vi "IMAQdx_Cam4.vi"(0 "Ctl Ref Record":refnum<vi>, 1 "Ctl Ref Cam":refnum<vi>, 2 "Session In":T6, 3 "Ctl Ref Folder":refnum<vi>, 5 "Cluster Buffer":T1={"Number of Images"=30, "Number of Workers"=5, "Skip Count"=0} {"Number of Workers" min=1 max=5}, 7 "Ctl Ref Time":refnum<vi>, 9 "Ctl Ref WriteSpeed":refnum<vi>, 11 "Ctl Ref Frames":refnum<vi>, 13 "Ctl Ref Stop":refnum<vi>) -> ()   [LabVIEW 2020]
uses:
  <vilib>/vision/driver/IMAQdx.llb/IMAQdx Acquisition Mode.ctl
  <vilib>/vision/Image Controls.llb/IMAQ Image.ctl
  <vilib>/vision/driver/IMAQdx.llb/IMAQdx Buffer Number Mode.ctl
  <vilib>/Utility/High Resolution Relative Seconds.vi
  <vilib>/functionblocks/Edge Detection/One Shot Rising with Input/One Shot Rising with Input.vi
  <vilib>/functionblocks/FB Core/FB Core.xnode
  <vilib>/vision/driver/NI_Vision_Acquisition_Software.lvlib
  <resource>/objmgr/imaqdx.rc
  <vilib>/functionblocks/NI_FunctionBlock Libraries.lvlib
panel:
  out "Cluster Frames":T2
  out "Cluster WriteSpeed":T3 {"WriteSpeed Worker5" format="%_19f"; "WriteSpeed Worker4" format="%_19f"; "WriteSpeed Worker3" format="%_19f"; "WriteSpeed Worker2" format="%_19f"; "WriteSpeed Worker1" format="%_19f"}
  out "Cluster BufferNr":T4
  out "Cluster LoopTimer":T5
  in  "Recording":bool
  out "VideoMode Camera":u32[](array[numeric])
  out "VideoMode Camera":string[](array[string])
  in  "Stop":bool
  out "Images in Queue":i32
  out "Camera":T7(plugin-control)
  out "LostBufferCount":u32
  out "Destination Folder":path
  in  "Stopped":bool
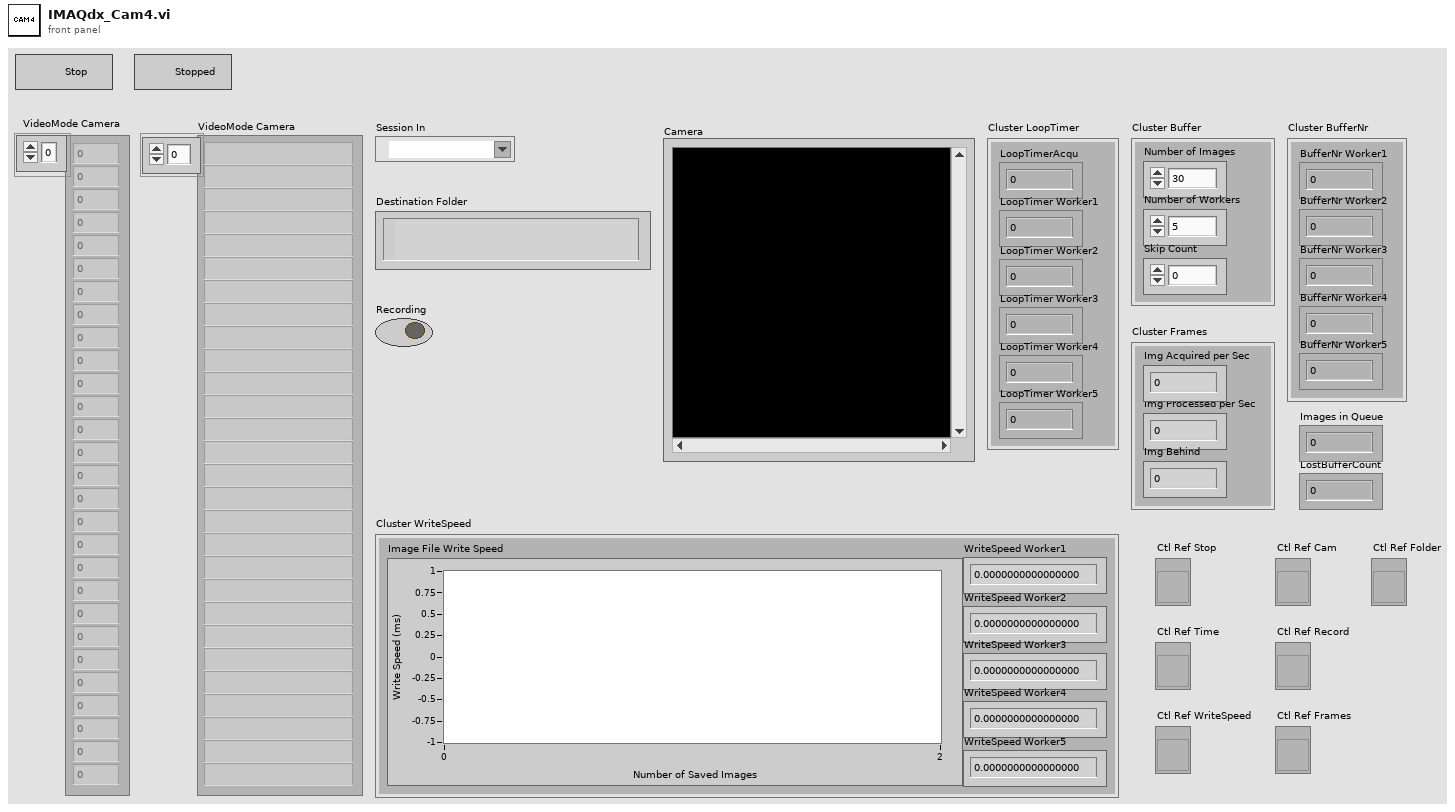
[diagram p1: front panel]
types:
  T1 = cluster{"Number of Images":i32, "Number of Workers":u8, "Skip Count":u32}
  T2 = cluster{"Img Processed per Sec":dbl, "Img Behind":i32, "Img Acquired per Sec":dbl}
  T3 = cluster{"WriteSpeed Worker1":dbl, "WriteSpeed Worker2":dbl, "WriteSpeed Worker3":dbl, "WriteSpeed Worker4":dbl, "WriteSpeed Worker5":dbl, "Write Speed":dbl}
  T4 = cluster{"BufferNr Worker1":u32, "BufferNr Worker2":u32, "BufferNr Worker3":u32, "BufferNr Worker4":u32, "BufferNr Worker5":u32}
  T5 = cluster{"LoopTimerAcqu":u32, "LoopTimer Worker1":u32, "LoopTimer Worker2":u32, "LoopTimer Worker3":u32, "LoopTimer Worker4":u32, "LoopTimer Worker5":u32}
  T6 = typedef "IMAQdx.ctl" = refnum<k21>
  T7 = typedef "IMAQ Image.ctl" = refnum<image>
  T8 = cluster{"Image Out":T7, "Buffer Number Out":u32, string}
  T9 = typedef "NI_Vision_Acquisition_Software.lvlib/IMAQdx Acquisition Mode.ctl" = enum32{"One Shot", "Continuous"}
  T10 = cluster{"Video Mode":u32, "Video Mode Name":string}[]
  T11 = typedef "NI_Vision_Acquisition_Software.lvlib/IMAQdx Buffer Number Mode.ctl" = enum32{"Next", "Last", "Buffer Number", "Every", "Last New"}
  T12 = cluster{"Image Out":T7, "Buffer Number Out":u32, "date/time string":string}
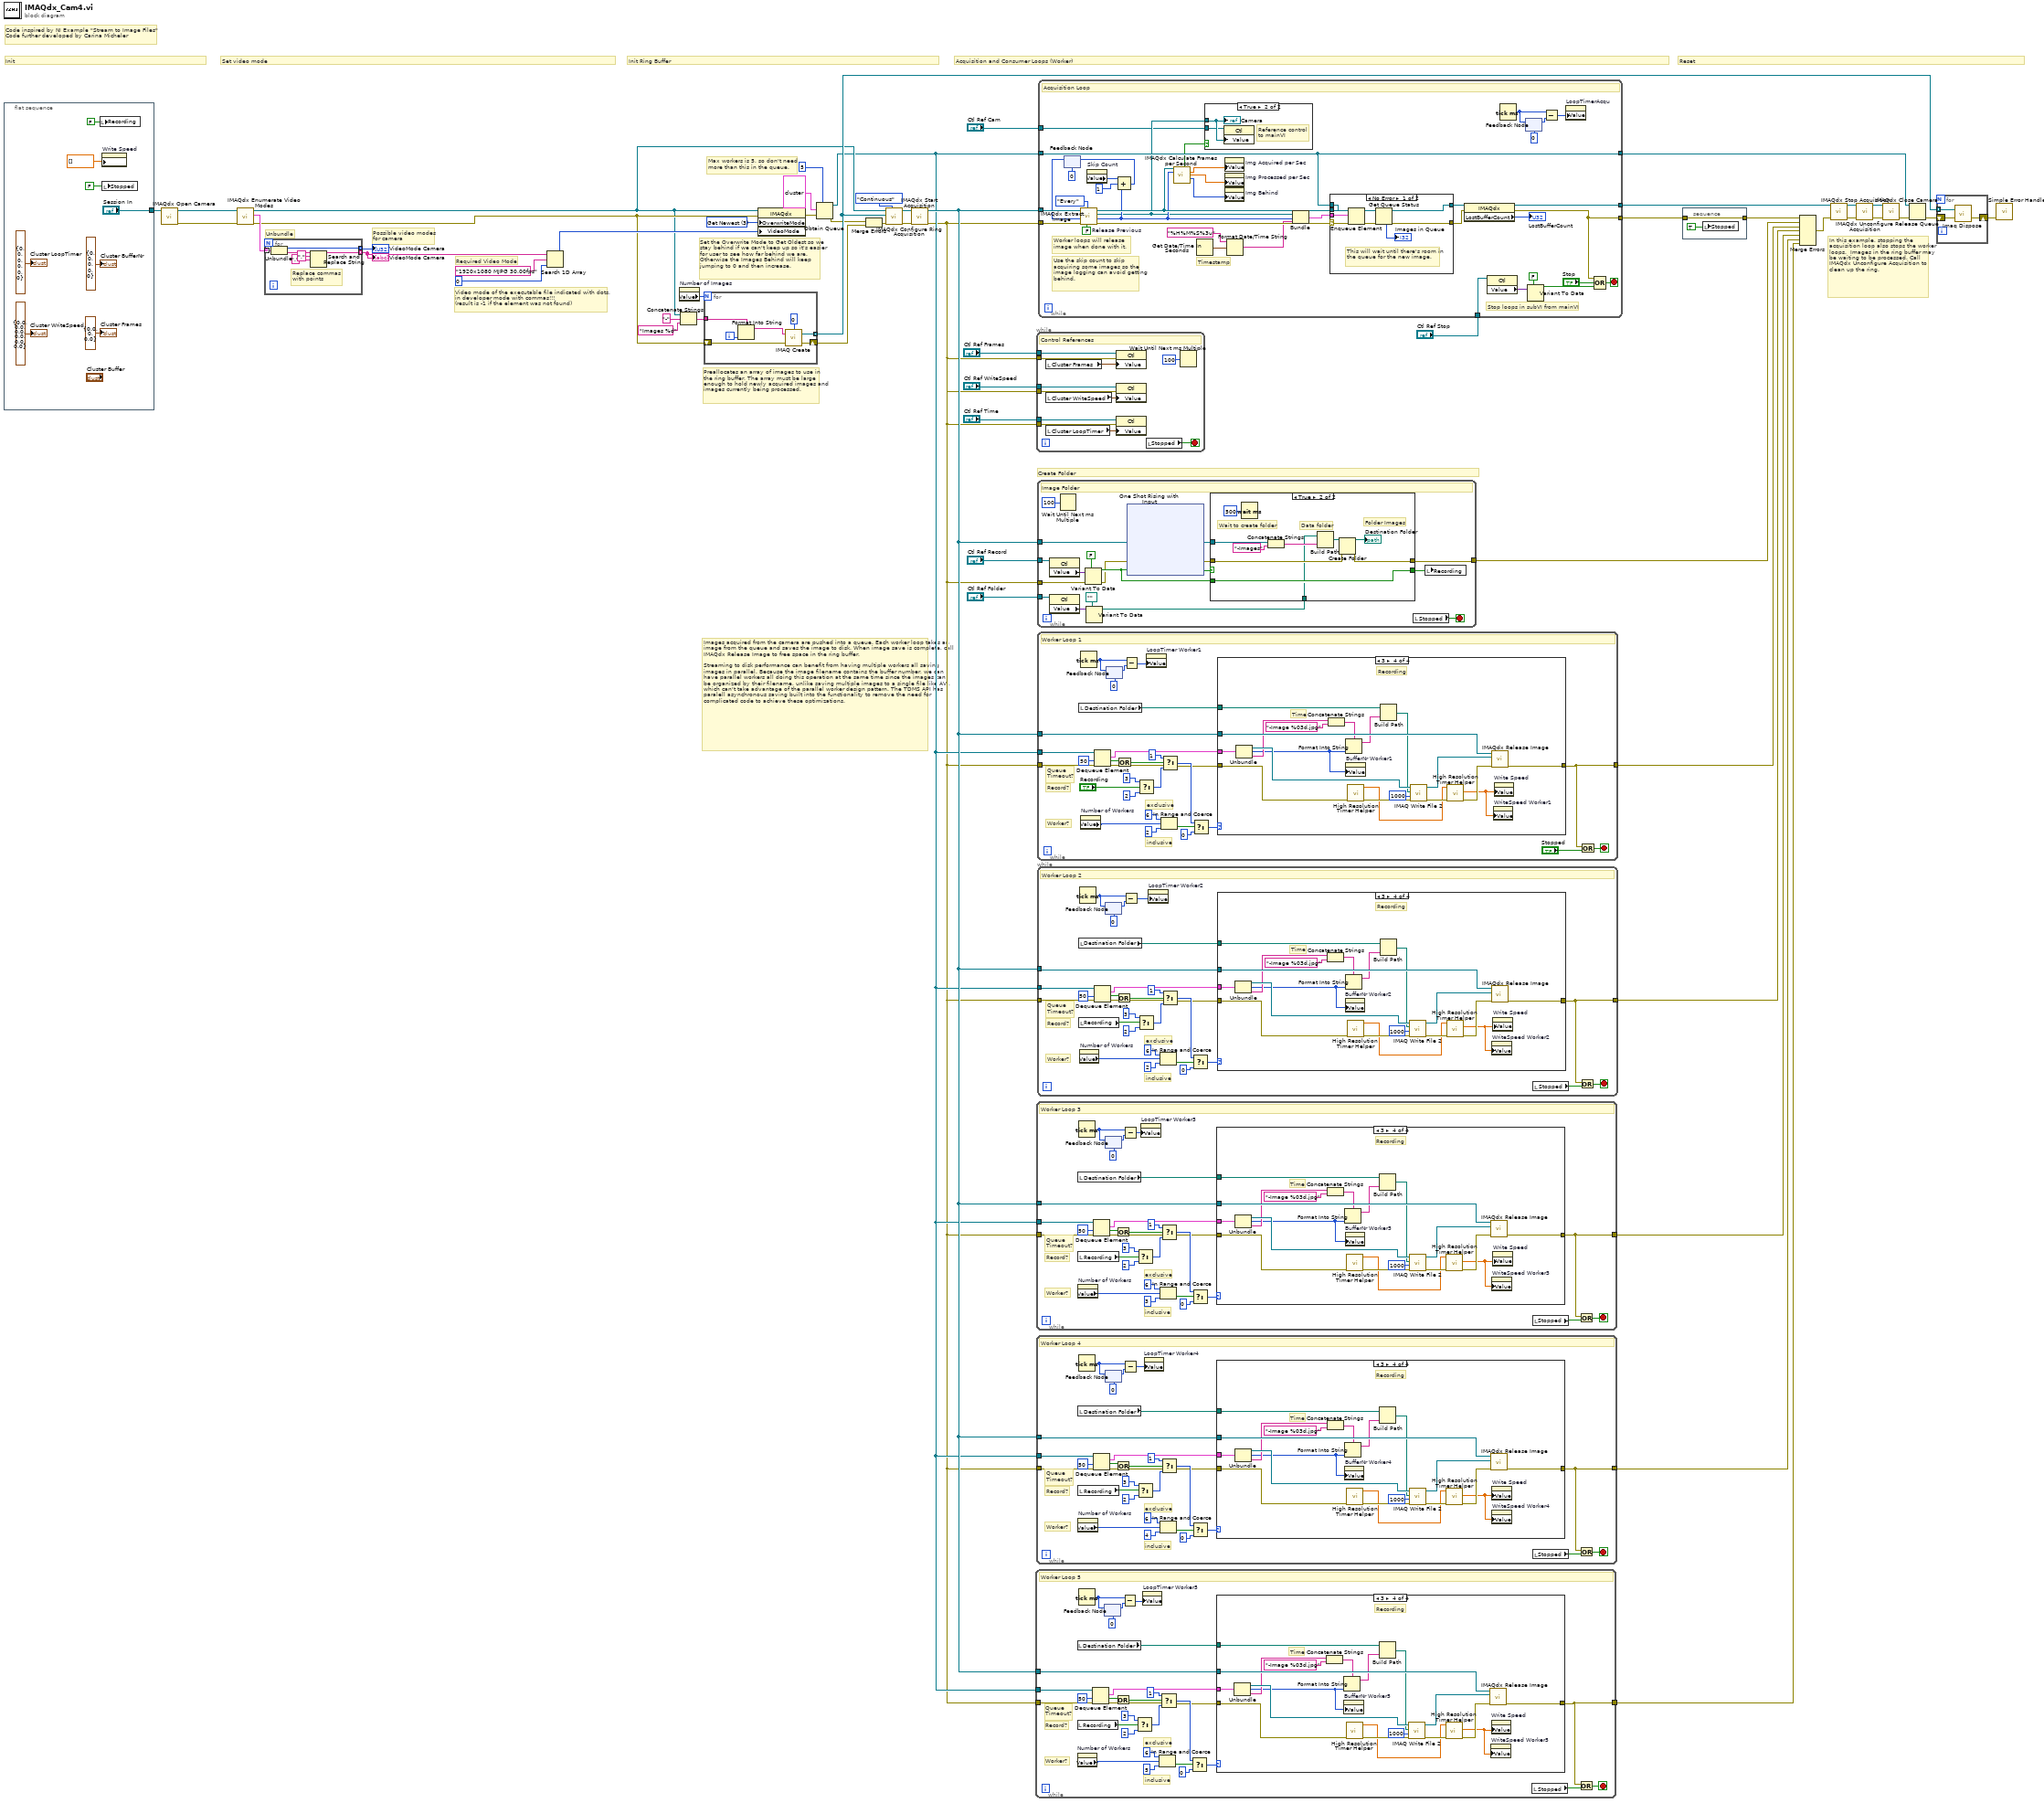
[diagram p0: block diagram]
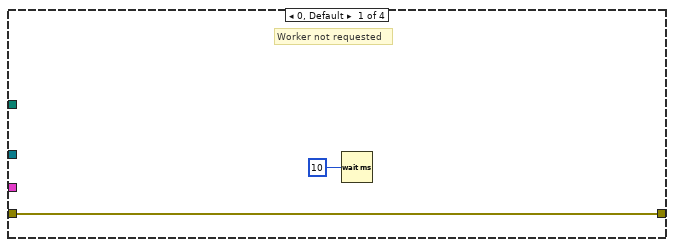
[diagram p2: hidden frame]
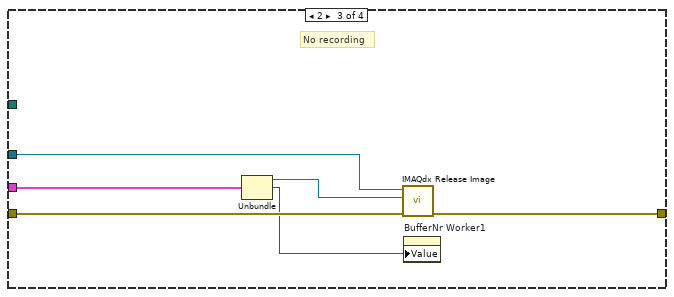
[diagram p4: hidden frame]
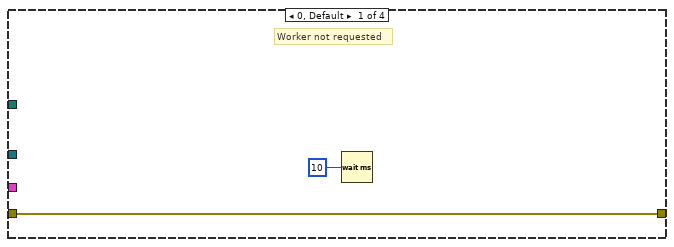
[diagram p5: hidden frame]
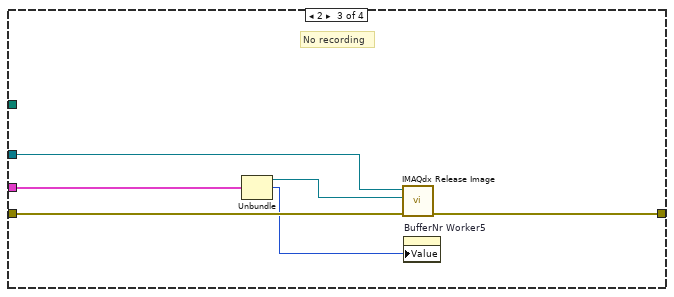
[diagram p7: hidden frame]
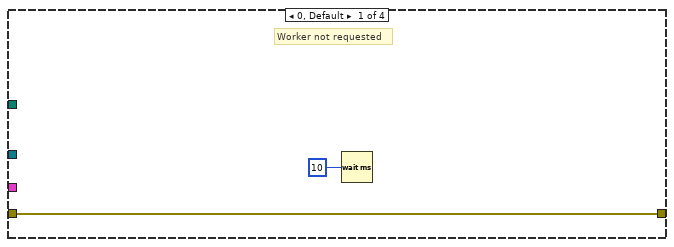
[diagram p8: hidden frame]
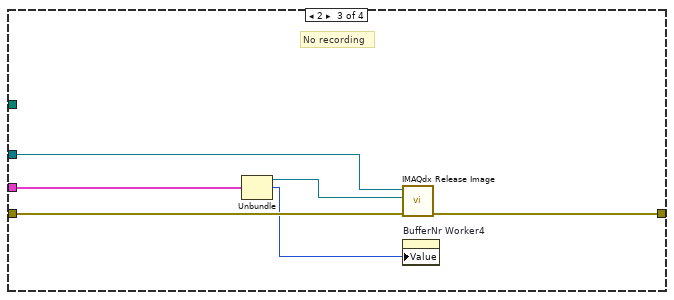
[diagram p10: hidden frame]
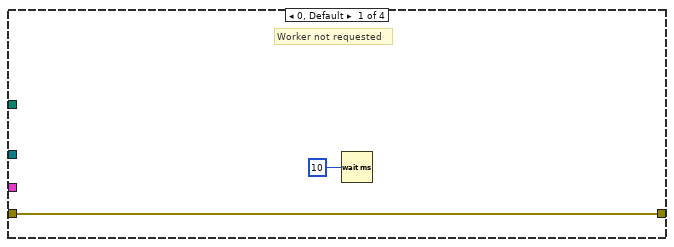
[diagram p11: hidden frame]
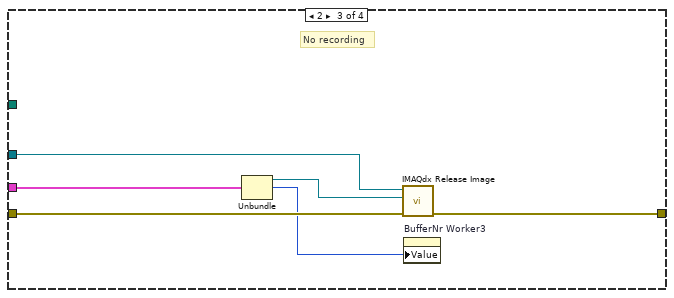
[diagram p13: hidden frame]
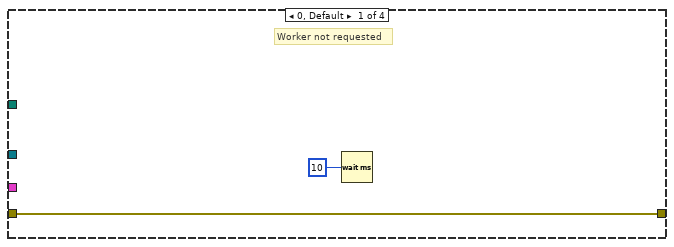
[diagram p15: hidden frame]
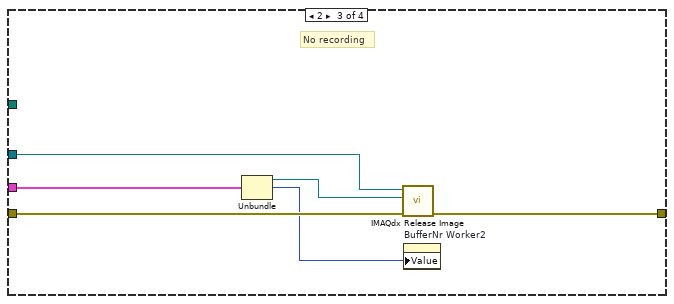
[diagram p17: hidden frame]
diagram:
  w35 = u32 3 items=["Get Oldest"=0, "Fail"=2, "Get Newest"=3] ("OverwriteMode")
  # "Create Folder"
  # "Images acquired from the camera are pushed into a queue. Each worker loop takes an image from the queue and saves the image to disk. When image save is complete, call IMAQdx Release Image to free space in the ring buffer. \n\nStreaming to disk performance can benefit from having multiple workers all saving images in parallel. Because the image filename contains the buffer number, we can have parallel workers all doing this operation at the same time since the images can be organized by their filename, unlike saving multiple images to a single file like AVI, which can't take advantage of the parallel worker design pattern. The TDMS API has paralell asynchronous saving built into the functionality to remove the need for complicated code to achieve these optimizations."
  # "Acquisition and Consumer Loops (Worker)"
  # "Reset"
  # "Code inspired by NI Example \"Stream to Image Files\"\nCode further developed by Carina Micheler"
  # "Init Ring Buffer"
  # "Init"
  # "Set video mode"
  # "Video mode of the executable file indicated with dots,\nin developer mode with commas!!!\n(result is -1 if the element was not found)"
  # "Required Video Mode"
  # "Possible video modes\nfor camera"
  # "Unbundle"
  # "Set the Overwrite Mode to Get Oldest so we stay behind if we can't keep up so it's easier for user to see how far behind we are. Otherwise the Images Behind will keep jumping to 0 and then increase."
  # "Max workers is 5, so don't need more than this in the queue."
  # "In this example, stopping the acquisition loop also stops the worker loops.  Images in the ring buffer may be waiting to be processed. Call IMAQdx Unconfigure Acquisition to clean up the ring."
  # "Preallocates an array of images to use in the ring buffer. The array must be large enough to hold newly acquired images and images currently being processed."
  n1 = flat-sequence {
    tunnel: ["Session In"] -> w22
    frame #0 {
      n2 = local write "Recording"(FALSE ("Recording")) -> ()
      n3 = property on="Write Speed" class="WFChart (strict)"("History Data"=dbl[] []) -> ()  [unwired: 2 in, 2 out]
      n4 = local write "Stopped"(FALSE ("Stop")) -> ()
      "Cluster LoopTimer" <- T5 {"LoopTimerAcqu"=0, "LoopTimer Worker1"=0, "LoopTimer Worker2"=0, "LoopTimer Worker3"=0, "LoopTimer Worker4"=0, "LoopTimer Worker5"=0} ("Cluster LoopTimer")
      "Cluster BufferNr" <- T4 {"BufferNr Worker1"=0, "BufferNr Worker2"=0, "BufferNr Worker3"=0, "BufferNr Worker4"=0, "BufferNr Worker5"=0} ("Cluster BufferNr")
      "Cluster WriteSpeed" <- T3 {"WriteSpeed Worker1"=0.0, "WriteSpeed Worker2"=0.0, "WriteSpeed Worker3"=0.0, "WriteSpeed Worker4"=0.0, "WriteSpeed Worker5"=0.0, "Write Speed"=0.0} ("Cluster WriteSpeed")
      "Cluster Frames" <- T2 {"Img Processed per Sec"=0.0, "Img Behind"=0, "Img Acquired per Sec"=0.0} ("Cluster Frames")
    }
  }
  n5 = call <vilib>:"IMAQdx Open Camera.vi"("Session In"=w22) -> ("error out"=w23:errorcluster, "Session Out"=w24:T6)  [unwired: 2 in, 7 out]
  n6 = call <vilib>:"IMAQdx Enumerate Video Modes.vi"("error in"=w23, "Session In"=w24) -> ("error out"=w25:errorcluster, "Video Modes"=w31:T10, "Session Out"=w15:T6)  [unwired: 6 in, 1 out]
  n7 = for {
    tunnel: w31 -> [w68] mode=indexing
    tunnel: [w67] -> w29 mode=indexing
    tunnel: [w63] -> w30 mode=indexing
    # "Replace commas \nwith points"
    n8 = Unbundle(w68) -> ("Video Mode"=w67:u32, "Video Mode Name"=w66:string)
    n9 = Search and Replace String(input string=w66, search string=",", replace string="." ("replace string (\"\")")) -> (result string=w63:string)  [unwired: 5 in, 3 out]
  }
  "VideoMode Camera" <- w30
  "VideoMode Camera" <- w29
  n10 = Search 1D Array(1D array=w30, element="1920x1080 MJPG 30.00fps", start index (0)=0) -> (index of element=w26:i32)
  n11 = property on="Number of Images" class="DigNum (strict)"() -> ("Value"=w7:i32)  [unwired: 2 in, 2 out]
  n12 = Concatenate Strings(w15, "-" ("string"), "Images %d" ("Image Name")) -> (w18:string)
  n13 = for {
    N: w7 -> [_]
    tunnel: [w74] -> w43 mode=indexing
    shift-right: [w73] -> w21
    shift-left: w25 -> [w75]
    tunnel: w18 -> [w69]
    i -> [w72]
    n14 = Format Into String(format string=w69, w72) -> (resulting string=w70:string)  [unwired: 2 in, 1 out]
    n15 = call "IMAQ Create"("Border Size"=0, "Image Name"=w70, "error in (no error)"=w75) -> ("New Image"=w74:T7, "error out"=w73:errorcluster)  [unwired: 1 in, 1 out]
  }
  n16 = property class="IMAQdx"(reference=w15, error in=w25, "OverwriteMode"=w35, "VideoMode"=w26) -> (error out=w34:errorcluster)  [unwired: 1 out]
  n17 = Obtain Queue(max queue size (-1, unlimited)=5, element data type=T8 {"Image Out"=refnum, "Buffer Number Out"=0, ""}, error in (no error)=w34) -> (queue out=w9:refnum<queue>, error out=w33:errorcluster)  [unwired: 2 in, 1 out]
  n18 = Merge Errors(w33, w21) -> (w46:errorcluster)
  n19 = call <vilib>:"IMAQdx Configure Ring Acquisition.vi"("Mode"=IMAQdx_Acquisition_Mode."Continuous" ("Continuous?"), "error in"=w46, "Images"=w43, "Session In"=w15) -> ("error out"=w49:errorcluster, "Session Out"=w50:T6)  [unwired: 5 in, 1 out]
  n20 = call <vilib>:"IMAQdx Start Acquisition.vi"("error in"=w49, "Session In"=w50) -> ("error out"=w3:errorcluster, "Session Out"=w10:T6)  [unwired: 8 out]
  n21 = while {
    tunnel: w9 -> [w80]
    tunnel: w10 -> [w102]
    tunnel: w3 -> [w82]
    tunnel: [w101] -> w11
    stop <- w103 stop-if-true
    # "Queue \nTimeout?"
    # "Record?"
    # "Worker?"
    # "inclusive"
    # "exclusive"
    # "Worker Loop 5"
    n22 = local read "Destination Folder"() -> (w99:path)
    n23 = local read "Recording"() -> (w93:bool)
    n24 = property on="Number of Workers" class="DigNum (strict)"() -> ("Value"=w76:u8)  [unwired: 2 in, 2 out]
    n25 = Tick Count (ms)() -> (millisecond timer value=w98:u32)
    n26 = Dequeue Element(queue=w80, timeout in ms (-1)=50 ("timeout in ms"), error in (no error)=w82) -> (element=w79:T8, timed out?=w90:bool, error out=w81:errorcluster)  [unwired: 1 out]
    n27 = feedback #1(u32 0 ("millisecond timer value")) -> (w97:u32)
    n28 = feedback-in #1(w98) -> ()
    n29 = Or(x=w90, y=w81) -> (x .or. y?=w92:bool)
    n30 = Subtract(x=w98, y=w97) -> (x-y=w77:u32)
    n31 = Select(t=u8 3 ("y"), s=w93, f=u8 2 ("y")) -> (s? t:f=w94:u8)
    n32 = property on="LoopTimer Worker5" class="DigNum (strict)"("Value"=w77) -> ()  [unwired: 2 in, 2 out]
    n33 = In Range and Coerce(upper limit=u8 6 ("y"), x=w76, lower limit=u8 5 ("y")) -> (In Range?=w95:bool)  [unwired: 1 out]
    n34 = Select(t=u8 1 ("y"), s=w92, f=w94) -> (s? t:f=w91:u8)
    n35 = Select(t=w91, s=w95, f=u8 0 ("y")) -> (s? t:f=w83:u8)
    n36 = case shown="3" w83 {
      tunnel: w102 -> [_ _ w112 w131]
      tunnel: w99 -> [_ _ _ w130]
      tunnel: w81 -> [w105 w106 w109 w128]
      tunnel: [w105 w106 w111 w129] -> w101
      tunnel: w79 -> [_ _ w110 w127]
      frame 0, Default {
        # "Worker not requested"
        n37 = Wait (ms)(milliseconds to wait=u32 10) -> ()  [unwired: 1 out]
      }
      frame 1 {
        # "Empty queue or error.\nNothing to process."
      }
      frame 2 {
        # "No recording"
        n38 = Unbundle(w110) -> ("Image Out"=w108:T7, "Buffer Number Out"=w107:u32)  [unwired: 1 out]
        n39 = call <vilib>:"IMAQdx Release Image.vi"("error in"=w109, "Image"=w108, "Session In"=w112) -> ("error out"=w111:errorcluster)  [unwired: 7 in, 1 out]
        n40 = property on="BufferNr Worker5" class="DigNum (strict)"("Value"=w107) -> ()  [unwired: 2 in, 2 out]
      }
      frame 3 {
        # "Recording"
        # "Time"
        n41 = Unbundle(w127) -> ("Image Out"=w126:T7, "Buffer Number Out"=w114:u32, w119:string)
        n42 = Concatenate Strings(w119, "-Image %03d.jpg" ("format string")) -> (w121:string)
        n43 = Format Into String(format string=w121, w114) -> (resulting string=w124:string)  [unwired: 2 in, 1 out]
        n44 = property on="BufferNr Worker5" class="DigNum (strict)"("Value"=w114) -> ()  [unwired: 2 in, 2 out]
        n45 = call "High Resolution Timer Helper.vi"("error in (no error)"=w128) -> ("error out"=w118:errorcluster, "Current Time"=w116:dbl)  [unwired: 8 in, 1 out]
        n46 = Build Path(base path=w130, name or relative path=w124) -> (appended path=w123:path)
        n47 = call-poly "IMAQ Write File 2"("error in (no error)"=w118, "Image Quality"=u32 1000, "File Path"=w123, "Image"=w126) -> ("error out"=w117:errorcluster, "Image Out (duplicate)"=w125:T7)  [unwired: 6 in]
        n48 = call "High Resolution Timer Helper.vi"("error in (no error)"=w117, "Previous Time"=w116) -> ("error out"=w122:errorcluster, "Time Difference (ms)"=w113:dbl)  [unwired: 7 in, 1 out]
        n49 = call <vilib>:"IMAQdx Release Image.vi"("error in"=w122, "Image"=w125, "Session In"=w131) -> ("error out"=w129:errorcluster)  [unwired: 7 in, 1 out]
        n50 = property on="WriteSpeed Worker5" class="DigNum (strict)"("Value"=w113) -> ()  [unwired: 2 in, 2 out]
        n51 = property on="Write Speed" class="WFChart (strict)"("Value"=w113) -> ()  [unwired: 2 in, 2 out]
      }
    }
    n52 = local read "Stopped"() -> (w100:bool)
    n53 = Or(x=w101, y=w100) -> (x .or. y?=w103:bool)
  }
  n54 = while {
    tunnel: "Ctl Ref Time" -> [w141]
    tunnel: w3 -> [w139]
    tunnel: "Ctl Ref WriteSpeed" -> [w136]
    tunnel: w3 -> [w137]
    tunnel: "Ctl Ref Frames" -> [w134]
    tunnel: w3 -> [w133]
    stop <- w140 stop-if-true
    # "Control References"
    n55 = local read "Cluster Frames"() -> (w132:T2)
    n56 = local read "Cluster WriteSpeed"() -> (w135:T3)
    n57 = local read "Cluster LoopTimer"() -> (w142:T5)
    n58 = property class="Ctl"(reference=w134, error in=w133, "Value"=w132) -> ()  [unwired: 2 out]
    n59 = property class="Ctl"(reference=w136, error in=w137, "Value"=w135) -> ()  [unwired: 2 out]
    n60 = property class="Ctl"(reference=w141, error in=w139, "Value"=w142) -> ()  [unwired: 2 out]
    n61 = local read "Stopped"() -> (w140:bool)
    n62 = Wait Until Next ms Multiple(millisecond multiple=u32 100) -> ()  [unwired: 1 out]
  }
  n63 = while {
    tunnel: w9 -> [w147]
    tunnel: w10 -> [w169]
    tunnel: w3 -> [w149]
    tunnel: [w168] -> w13
    stop <- w170 stop-if-true
    # "Queue \nTimeout?"
    # "Record?"
    # "Worker?"
    # "inclusive"
    # "exclusive"
    # "Worker Loop 3"
    n64 = local read "Destination Folder"() -> (w166:path)
    n65 = local read "Recording"() -> (w160:bool)
    n66 = property on="Number of Workers" class="DigNum (strict)"() -> ("Value"=w143:u8)  [unwired: 2 in, 2 out]
    n67 = Tick Count (ms)() -> (millisecond timer value=w165:u32)
    n68 = Dequeue Element(queue=w147, timeout in ms (-1)=50 ("timeout in ms"), error in (no error)=w149) -> (element=w146:T8, timed out?=w157:bool, error out=w148:errorcluster)  [unwired: 1 out]
    n69 = feedback #2(u32 0 ("millisecond timer value")) -> (w164:u32)
    n70 = feedback-in #2(w165) -> ()
    n71 = Or(x=w157, y=w148) -> (x .or. y?=w159:bool)
    n72 = Subtract(x=w165, y=w164) -> (x-y=w144:u32)
    n73 = Select(t=u8 3 ("y"), s=w160, f=u8 2 ("y")) -> (s? t:f=w161:u8)
    n74 = property on="LoopTimer Worker3" class="DigNum (strict)"("Value"=w144) -> ()  [unwired: 2 in, 2 out]
    n75 = In Range and Coerce(upper limit=u8 6 ("y"), x=w143, lower limit=u8 3 ("y")) -> (In Range?=w162:bool)  [unwired: 1 out]
    n76 = Select(t=u8 1 ("y"), s=w159, f=w161) -> (s? t:f=w158:u8)
    n77 = Select(t=w158, s=w162, f=u8 0 ("y")) -> (s? t:f=w150:u8)
    n78 = case shown="3" w150 {
      tunnel: w169 -> [_ _ w179 w198]
      tunnel: w166 -> [_ _ _ w197]
      tunnel: w148 -> [w172 w173 w176 w195]
      tunnel: [w172 w173 w178 w196] -> w168
      tunnel: w146 -> [_ _ w177 w194]
      frame 0, Default {
        # "Worker not requested"
        n79 = Wait (ms)(milliseconds to wait=u32 10) -> ()  [unwired: 1 out]
      }
      frame 1 {
        # "Empty queue or error.\nNothing to process."
      }
      frame 2 {
        # "No recording"
        n80 = Unbundle(w177) -> ("Image Out"=w175:T7, "Buffer Number Out"=w174:u32)  [unwired: 1 out]
        n81 = call <vilib>:"IMAQdx Release Image.vi"("error in"=w176, "Image"=w175, "Session In"=w179) -> ("error out"=w178:errorcluster)  [unwired: 7 in, 1 out]
        n82 = property on="BufferNr Worker3" class="DigNum (strict)"("Value"=w174) -> ()  [unwired: 2 in, 2 out]
      }
      frame 3 {
        # "Recording"
        # "Time"
        n83 = Unbundle(w194) -> ("Image Out"=w193:T7, "Buffer Number Out"=w181:u32, w186:string)
        n84 = Concatenate Strings(w186, "-Image %03d.jpg" ("format string")) -> (w188:string)
        n85 = Format Into String(format string=w188, w181) -> (resulting string=w191:string)  [unwired: 2 in, 1 out]
        n86 = property on="BufferNr Worker3" class="DigNum (strict)"("Value"=w181) -> ()  [unwired: 2 in, 2 out]
        n87 = call "High Resolution Timer Helper.vi"("error in (no error)"=w195) -> ("error out"=w185:errorcluster, "Current Time"=w183:dbl)  [unwired: 8 in, 1 out]
        n88 = Build Path(base path=w197, name or relative path=w191) -> (appended path=w190:path)
        n89 = call-poly "IMAQ Write File 2"("error in (no error)"=w185, "Image Quality"=u32 1000, "File Path"=w190, "Image"=w193) -> ("error out"=w184:errorcluster, "Image Out (duplicate)"=w192:T7)  [unwired: 6 in]
        n90 = call "High Resolution Timer Helper.vi"("error in (no error)"=w184, "Previous Time"=w183) -> ("error out"=w189:errorcluster, "Time Difference (ms)"=w180:dbl)  [unwired: 7 in, 1 out]
        n91 = call <vilib>:"IMAQdx Release Image.vi"("error in"=w189, "Image"=w192, "Session In"=w198) -> ("error out"=w196:errorcluster)  [unwired: 7 in, 1 out]
        n92 = property on="WriteSpeed Worker3" class="DigNum (strict)"("Value"=w180) -> ()  [unwired: 2 in, 2 out]
        n93 = property on="Write Speed" class="WFChart (strict)"("Value"=w180) -> ()  [unwired: 2 in, 2 out]
      }
    }
    n94 = local read "Stopped"() -> (w167:bool)
    n95 = Or(x=w168, y=w167) -> (x .or. y?=w170:bool)
  }
  n96 = while {
    tunnel: w9 -> [w203]
    tunnel: w10 -> [w225]
    tunnel: w3 -> [w205]
    tunnel: [w224] -> w12
    stop <- w226 stop-if-true
    # "Queue \nTimeout?"
    # "Record?"
    # "Worker?"
    # "inclusive"
    # "exclusive"
    # "Worker Loop 4"
    n97 = local read "Destination Folder"() -> (w222:path)
    n98 = local read "Recording"() -> (w216:bool)
    n99 = property on="Number of Workers" class="DigNum (strict)"() -> ("Value"=w199:u8)  [unwired: 2 in, 2 out]
    n100 = Tick Count (ms)() -> (millisecond timer value=w221:u32)
    n101 = Dequeue Element(queue=w203, timeout in ms (-1)=50 ("timeout in ms"), error in (no error)=w205) -> (element=w202:T8, timed out?=w213:bool, error out=w204:errorcluster)  [unwired: 1 out]
    n102 = feedback #3(u32 0 ("millisecond timer value")) -> (w220:u32)
    n103 = feedback-in #3(w221) -> ()
    n104 = Or(x=w213, y=w204) -> (x .or. y?=w215:bool)
    n105 = Subtract(x=w221, y=w220) -> (x-y=w200:u32)
    n106 = Select(t=u8 3 ("y"), s=w216, f=u8 2 ("y")) -> (s? t:f=w217:u8)
    n107 = property on="LoopTimer Worker4" class="DigNum (strict)"("Value"=w200) -> ()  [unwired: 2 in, 2 out]
    n108 = In Range and Coerce(upper limit=u8 6 ("y"), x=w199, lower limit=u8 4 ("y")) -> (In Range?=w218:bool)  [unwired: 1 out]
    n109 = Select(t=u8 1 ("y"), s=w215, f=w217) -> (s? t:f=w214:u8)
    n110 = Select(t=w214, s=w218, f=u8 0 ("y")) -> (s? t:f=w206:u8)
    n111 = case shown="3" w206 {
      tunnel: w225 -> [_ _ w235 w254]
      tunnel: w222 -> [_ _ _ w253]
      tunnel: w204 -> [w228 w229 w232 w251]
      tunnel: [w228 w229 w234 w252] -> w224
      tunnel: w202 -> [_ _ w233 w250]
      frame 0, Default {
        # "Worker not requested"
        n112 = Wait (ms)(milliseconds to wait=u32 10) -> ()  [unwired: 1 out]
      }
      frame 1 {
        # "Empty queue or error.\nNothing to process."
      }
      frame 2 {
        # "No recording"
        n113 = Unbundle(w233) -> ("Image Out"=w231:T7, "Buffer Number Out"=w230:u32)  [unwired: 1 out]
        n114 = call <vilib>:"IMAQdx Release Image.vi"("error in"=w232, "Image"=w231, "Session In"=w235) -> ("error out"=w234:errorcluster)  [unwired: 7 in, 1 out]
        n115 = property on="BufferNr Worker4" class="DigNum (strict)"("Value"=w230) -> ()  [unwired: 2 in, 2 out]
      }
      frame 3 {
        # "Recording"
        # "Time"
        n116 = Unbundle(w250) -> ("Image Out"=w249:T7, "Buffer Number Out"=w237:u32, w242:string)
        n117 = Concatenate Strings(w242, "-Image %03d.jpg" ("format string")) -> (w244:string)
        n118 = Format Into String(format string=w244, w237) -> (resulting string=w247:string)  [unwired: 2 in, 1 out]
        n119 = property on="BufferNr Worker4" class="DigNum (strict)"("Value"=w237) -> ()  [unwired: 2 in, 2 out]
        n120 = call "High Resolution Timer Helper.vi"("error in (no error)"=w251) -> ("error out"=w241:errorcluster, "Current Time"=w239:dbl)  [unwired: 8 in, 1 out]
        n121 = Build Path(base path=w253, name or relative path=w247) -> (appended path=w246:path)
        n122 = call-poly "IMAQ Write File 2"("error in (no error)"=w241, "Image Quality"=u32 1000, "File Path"=w246, "Image"=w249) -> ("error out"=w240:errorcluster, "Image Out (duplicate)"=w248:T7)  [unwired: 6 in]
        n123 = call "High Resolution Timer Helper.vi"("error in (no error)"=w240, "Previous Time"=w239) -> ("error out"=w245:errorcluster, "Time Difference (ms)"=w236:dbl)  [unwired: 7 in, 1 out]
        n124 = call <vilib>:"IMAQdx Release Image.vi"("error in"=w245, "Image"=w248, "Session In"=w254) -> ("error out"=w252:errorcluster)  [unwired: 7 in, 1 out]
        n125 = property on="Write Speed" class="WFChart (strict)"("Value"=w236) -> ()  [unwired: 2 in, 2 out]
        n126 = property on="WriteSpeed Worker4" class="DigNum (strict)"("Value"=w236) -> ()  [unwired: 2 in, 2 out]
      }
    }
    n127 = local read "Stopped"() -> (w223:bool)
    n128 = Or(x=w224, y=w223) -> (x .or. y?=w226:bool)
  }
  n129 = while {
    tunnel: w9 -> [w258]
    tunnel: w10 -> [w281]
    tunnel: w3 -> [w260]
    tunnel: [w280] -> w37
    stop <- w282 stop-if-true
    # "Queue \nTimeout?"
    # "Record?"
    # "Worker?"
    # "inclusive"
    # "exclusive"
    # "Worker Loop 2"
    n130 = local read "Destination Folder"() -> (w278:path)
    n131 = local read "Recording"() -> (w272:bool)
    n132 = Tick Count (ms)() -> (millisecond timer value=w277:u32)
    n133 = property on="Number of Workers" class="DigNum (strict)"() -> ("Value"=w255:u8)  [unwired: 2 in, 2 out]
    n134 = Dequeue Element(queue=w258, timeout in ms (-1)=50 ("timeout in ms"), error in (no error)=w260) -> (element=w257:T8, timed out?=w269:bool, error out=w259:errorcluster)  [unwired: 1 out]
    n135 = feedback #4(u32 0 ("millisecond timer value")) -> (w276:u32)
    n136 = feedback-in #4(w277) -> ()
    n137 = Or(x=w269, y=w259) -> (x .or. y?=w271:bool)
    n138 = Subtract(x=w277, y=w276) -> (x-y=w256:u32)
    n139 = Select(t=u8 3 ("y"), s=w272, f=u8 2 ("y")) -> (s? t:f=w273:u8)
    n140 = property on="LoopTimer Worker2" class="DigNum (strict)"("Value"=w256) -> ()  [unwired: 2 in, 2 out]
    n141 = In Range and Coerce(upper limit=u8 6 ("y"), x=w255, lower limit=u8 2 ("y")) -> (In Range?=w274:bool)  [unwired: 1 out]
    n142 = Select(t=u8 1 ("y"), s=w271, f=w273) -> (s? t:f=w270:u8)
    n143 = Select(t=w270, s=w274, f=u8 0 ("y")) -> (s? t:f=w261:u8)
    n144 = case shown="3" w261 {
      tunnel: w281 -> [_ _ w291 w310]
      tunnel: w278 -> [_ _ _ w309]
      tunnel: w259 -> [w284 w285 w288 w307]
      tunnel: [w284 w285 w290 w308] -> w280
      tunnel: w257 -> [_ _ w289 w306]
      frame 0, Default {
        # "Worker not requested"
        n145 = Wait (ms)(milliseconds to wait=u32 10) -> ()  [unwired: 1 out]
      }
      frame 1 {
        # "Empty queue or error.\nNothing to process."
      }
      frame 2 {
        # "No recording"
        n146 = Unbundle(w289) -> ("Image Out"=w287:T7, "Buffer Number Out"=w286:u32)  [unwired: 1 out]
        n147 = call <vilib>:"IMAQdx Release Image.vi"("error in"=w288, "Image"=w287, "Session In"=w291) -> ("error out"=w290:errorcluster)  [unwired: 7 in, 1 out]
        n148 = property on="BufferNr Worker2" class="DigNum (strict)"("Value"=w286) -> ()  [unwired: 2 in, 2 out]
      }
      frame 3 {
        # "Recording"
        # "Time"
        n149 = Unbundle(w306) -> ("Image Out"=w305:T7, "Buffer Number Out"=w293:u32, w298:string)
        n150 = Concatenate Strings(w298, "-Image %03d.jpg" ("format string")) -> (w300:string)
        n151 = Format Into String(format string=w300, w293) -> (resulting string=w303:string)  [unwired: 2 in, 1 out]
        n152 = property on="BufferNr Worker2" class="DigNum (strict)"("Value"=w293) -> ()  [unwired: 2 in, 2 out]
        n153 = call "High Resolution Timer Helper.vi"("error in (no error)"=w307) -> ("error out"=w297:errorcluster, "Current Time"=w295:dbl)  [unwired: 8 in, 1 out]
        n154 = Build Path(base path=w309, name or relative path=w303) -> (appended path=w302:path)
        n155 = call-poly "IMAQ Write File 2"("error in (no error)"=w297, "Image Quality"=u32 1000, "File Path"=w302, "Image"=w305) -> ("error out"=w296:errorcluster, "Image Out (duplicate)"=w304:T7)  [unwired: 6 in]
        n156 = call "High Resolution Timer Helper.vi"("error in (no error)"=w296, "Previous Time"=w295) -> ("error out"=w301:errorcluster, "Time Difference (ms)"=w292:dbl)  [unwired: 7 in, 1 out]
        n157 = call <vilib>:"IMAQdx Release Image.vi"("error in"=w301, "Image"=w304, "Session In"=w310) -> ("error out"=w308:errorcluster)  [unwired: 7 in, 1 out]
        n158 = property on="WriteSpeed Worker2" class="DigNum (strict)"("Value"=w292) -> ()  [unwired: 2 in, 2 out]
        n159 = property on="Write Speed" class="WFChart (strict)"("Value"=w292) -> ()  [unwired: 2 in, 2 out]
      }
    }
    n160 = local read "Stopped"() -> (w279:bool)
    n161 = Or(x=w280, y=w279) -> (x .or. y?=w282:bool)
  }
  n162 = while {
    tunnel: w10 -> [w327]
    tunnel: "Ctl Ref Record" -> [w322]
    tunnel: w3 -> [w314]
    tunnel: [w321] -> w2
    tunnel: "Ctl Ref Folder" -> [w315]
    stop <- w326 stop-if-true
    # "Image Folder"
    n163 = property class="Ctl"(reference=w322) -> ("Value"=w324:variant)  [unwired: 1 in, 2 out]
    n164 = property class="Ctl"(reference=w315) -> ("Value"=w313:variant)  [unwired: 1 in, 2 out]
    n165 = Wait Until Next ms Multiple(millisecond multiple=u32 100) -> ()  [unwired: 1 out]
    n166 = Variant To Data(error in=w314, type=FALSE, Variant=w324) -> (data=w320:bool, error out=w317:errorcluster)
    n167 = Variant To Data(type=path "" ("Path"), Variant=w313) -> (data=w311:path)  [unwired: 1 in, 1 out]
    n168 = xnode "One Shot Rising with Input"("error in"=w317, "input"=w320) -> ("error out"=w318:errorcluster, "output"=w319:bool)
    n169 = case shown="True" w319 {
      tunnel: w327 -> [_ w376]
      tunnel: [w367 w371] -> w321
      tunnel: w318 -> [w367 w370]
      tunnel: w320 -> [w366 w369]
      tunnel: [w366 w369] -> w316
      tunnel: w311 -> [_ w368]
      frame False {
      }
      frame True {
        # "Folder Images"
        # "Data folder"
        # "Wait to create folder"
        n170 = Wait (ms)(milliseconds to wait=u32 500) -> ()  [unwired: 1 out]
        n171 = Concatenate Strings(w376, "-Images" ("Folder Name")) -> (w373:string)
        n172 = Build Path(base path=w368, name or relative path=w373) -> (appended path=w374:path)
        n173 = Create Folder(path (use dialog)=w374, error in=w370) -> (created path=→"Destination Folder":path, error out=w371:errorcluster)  [unwired: 1 in, 1 out]
      }
    }
    n174 = local read "Stopped"() -> (w326:bool)
    n175 = local write "Recording"(w316) -> ()
  }
  n176 = while {
    tunnel: w9 -> [w383]
    tunnel: w10 -> [w404]
    tunnel: w3 -> [w385]
    tunnel: [w403] -> w8
    stop <- w405 stop-if-true
    # "Queue \nTimeout?"
    # "Record?"
    # "Worker?"
    # "inclusive"
    # "exclusive"
    # "Worker Loop 1"
    n177 = local read "Destination Folder"() -> (w402:path)
    n178 = Tick Count (ms)() -> (millisecond timer value=w401:u32)
    n179 = property on="Number of Workers" class="DigNum (strict)"() -> ("Value"=w378:u8)  [unwired: 2 in, 2 out]
    n180 = Dequeue Element(queue=w383, timeout in ms (-1)=50 ("timeout in ms"), error in (no error)=w385) -> (element=w382:T8, timed out?=w394:bool, error out=w384:errorcluster)  [unwired: 1 out]
    n181 = feedback #5(u32 0 ("millisecond timer value")) -> (w400:u32)
    n182 = feedback-in #5(w401) -> ()
    n183 = Or(x=w394, y=w384) -> (x .or. y?=w396:bool)
    n184 = Subtract(x=w401, y=w400) -> (x-y=w379:u32)
    n185 = Select(t=u8 3 ("y"), s="Recording", f=u8 2 ("y")) -> (s? t:f=w397:u8)
    n186 = property on="LoopTimer Worker1" class="DigNum (strict)"("Value"=w379) -> ()  [unwired: 2 in, 2 out]
    n187 = In Range and Coerce(upper limit=u8 6 ("y"), x=w378, lower limit=u8 2 ("y")) -> (In Range?=w398:bool)  [unwired: 1 out]
    n188 = Select(t=u8 1 ("y"), s=w396, f=w397) -> (s? t:f=w395:u8)
    n189 = Select(t=w395, s=w398, f=u8 0 ("y")) -> (s? t:f=w386:u8)
    n190 = case shown="3" w386 {
      tunnel: w404 -> [_ _ w414 w433]
      tunnel: w402 -> [_ _ _ w432]
      tunnel: w384 -> [w407 w408 w411 w430]
      tunnel: [w407 w408 w413 w431] -> w403
      tunnel: w382 -> [_ _ w412 w429]
      frame 0, Default {
        # "Worker not requested"
        n191 = Wait (ms)(milliseconds to wait=u32 10) -> ()  [unwired: 1 out]
      }
      frame 1 {
        # "Empty queue or error.\nNothing to process."
      }
      frame 2 {
        # "No recording"
        n192 = Unbundle(w412) -> ("Image Out"=w410:T7, "Buffer Number Out"=w409:u32)  [unwired: 1 out]
        n193 = call <vilib>:"IMAQdx Release Image.vi"("error in"=w411, "Image"=w410, "Session In"=w414) -> ("error out"=w413:errorcluster)  [unwired: 7 in, 1 out]
        n194 = property on="BufferNr Worker1" class="DigNum (strict)"("Value"=w409) -> ()  [unwired: 2 in, 2 out]
      }
      frame 3 {
        # "Recording"
        # "Time"
        n195 = Unbundle(w429) -> ("Image Out"=w428:T7, "Buffer Number Out"=w416:u32, w421:string)
        n196 = Concatenate Strings(w421, "-Image %03d.jpg" ("format string")) -> (w423:string)
        n197 = Format Into String(format string=w423, w416) -> (resulting string=w426:string)  [unwired: 2 in, 1 out]
        n198 = property on="BufferNr Worker1" class="DigNum (strict)"("Value"=w416) -> ()  [unwired: 2 in, 2 out]
        n199 = call "High Resolution Timer Helper.vi"("error in (no error)"=w430) -> ("error out"=w420:errorcluster, "Current Time"=w418:dbl)  [unwired: 8 in, 1 out]
        n200 = Build Path(base path=w432, name or relative path=w426) -> (appended path=w425:path)
        n201 = call-poly "IMAQ Write File 2"("error in (no error)"=w420, "Image Quality"=u32 1000, "File Path"=w425, "Image"=w428) -> ("error out"=w419:errorcluster, "Image Out (duplicate)"=w427:T7)  [unwired: 6 in]
        n202 = call "High Resolution Timer Helper.vi"("error in (no error)"=w419, "Previous Time"=w418) -> ("error out"=w424:errorcluster, "Time Difference (ms)"=w415:dbl)  [unwired: 7 in, 1 out]
        n203 = call <vilib>:"IMAQdx Release Image.vi"("error in"=w424, "Image"=w427, "Session In"=w433) -> ("error out"=w431:errorcluster)  [unwired: 7 in, 1 out]
        n204 = property on="WriteSpeed Worker1" class="DigNum (strict)"("Value"=w415) -> ()  [unwired: 2 in, 2 out]
        n205 = property on="Write Speed" class="WFChart (strict)"("Value"=w415) -> ()  [unwired: 2 in, 2 out]
      }
    }
    n206 = Or(x=w403, y="Stopped") -> (x .or. y?=w405:bool)
  }
  n207 = while {
    tunnel: w3 -> [w471]
    tunnel: w10 -> [w468]
    tunnel: w9 -> [w467]
    tunnel: [w454] -> w42
    tunnel: [w453] -> w39
    tunnel: [w467] -> w44
    tunnel: "Ctl Ref Stop" -> [w448]
    tunnel: "Ctl Ref Cam" -> [w447]
    stop <- w466 stop-if-true
    w469 = FALSE  # Release Previous
    # "Timestamp"
    # "Stop loops in subVI from mainVI"
    # "Use the skip count to skip acquiring some images so the image logging can avoid getting behind."
    # "Worker loops will release image when done with it."
    # "Acquisition Loop"
    n208 = feedback #6(u32 0) -> (w464:u32)
    n209 = call <vilib>:"IMAQdx Extract Image.vi"("Release Previous (true)"=w469, "Buffer Number Mode (Next)"=IMAQdx_Buffer_Number_Mode."Every" ("Buffer Number Mode"), "error in"=w471, "Buffer Number In"=w464, "Session In"=w468) -> ("error out"=w456:errorcluster, "Buffer Number Out"=w460:u32, "Image Out"=w455:T7, "Session Out"=w461:T6)  [unwired: 3 in]
    n210 = property on="Skip Count" class="DigNum (strict)"() -> ("Value"=w435:u32)  [unwired: 2 in, 2 out]
    n211 = Compound Arithmetic op=ADD(w435, u32 1 ("value"), w460) -> (w465:u32)
    n212 = feedback-in #6(w465) -> ()
    n213 = call <vilib>:"IMAQdx Calculate Frames per Second.vi"("Session In"=w461, "Buffer Number"=w460) -> ("Update Display"=w434:bool, "Acquired Frames per Second"=w438:dbl, "Processed Frames per Second"=w437:dbl, "Images Behind"=w436:i32)  [unwired: 7 in, 3 out]
    n214 = Get Date/Time In Seconds() -> (seconds since 1Jan1904=w445:timestamp)
    n215 = case shown="True" w434 {
      tunnel: w455 -> [_ w483]
      tunnel: w447 -> [_ w482]
      frame False {
      }
      frame True {
        # "Reference control\nto mainVI"
        n216 = property class="Ctl"(reference=w482, "Value"=w483) -> ()  [unwired: 1 in, 2 out]
        "Camera" <- w483
      }
    }
    n217 = property on="Img Acquired per Sec" class="DigNum (strict)"("Value"=w438) -> ()  [unwired: 2 in, 2 out]
    n218 = property on="Img Processed per Sec" class="DigNum (strict)"("Value"=w437) -> ()  [unwired: 2 in, 2 out]
    n219 = property on="Img Behind" class="DigNum (strict)"("Value"=w436) -> ()  [unwired: 2 in, 2 out]
    n220 = Format Date/Time String(time format string (%c)="%H%M%S%3u", seconds (now)=w445) -> (date/time string=w444:string)  [unwired: 1 in]
    n221 = Bundle("Image Out"=w455, "Buffer Number Out"=w460, "date/time string"=w444) -> (w446:T12)  [unwired: 1 in]
    n222 = case shown="No Error" w456 {
      selector: w456 -> [w479 w480]
      tunnel: [w477 w481] -> w442
      tunnel: w461 -> [w477 w481]
      tunnel: w446 -> [w476 _]
      tunnel: w467 -> [w478 _]
      tunnel: [w474 w480] -> w441
      frame No Error {
        # "This will wait until there's room in the queue for the new image."
        n223 = Enqueue Element(queue=w478, element=w476, error in (no error)=w479) -> (queue out=w473:refnum<queue>, error out=w475:errorcluster)  [unwired: 1 in, 1 out]
        n224 = Get Queue Status(queue=w473, error in (no error)=w475) -> (error out=w474:errorcluster, # elements in queue=→"Images in Queue":i32)  [unwired: 1 in, 6 out]
      }
      frame Error {
      }
    }
    n225 = property class="IMAQdx"(reference=w442, error in=w441) -> (reference out=w454:T6, error out=w453:errorcluster, "LostBufferCount"=→"LostBufferCount":u32)
    n226 = property class="Ctl"(reference=w448) -> ("Value"=w451:variant)  [unwired: 1 in, 2 out]
    n227 = Tick Count (ms)() -> (millisecond timer value=w459:u32)
    n228 = feedback #7(u32 0 ("millisecond timer value")) -> (w458:u32)
    n229 = feedback-in #7(w459) -> ()
    n230 = Variant To Data(type=FALSE, Variant=w451) -> (data=w449:bool)  [unwired: 1 in, 1 out]
    n231 = Subtract(x=w459, y=w458) -> (x-y=w439:u32)
    n232 = property on="LoopTimerAcqu" class="DigNum (strict)"("Value"=w439) -> ()  [unwired: 2 in, 2 out]
    n233 = Compound Arithmetic op=OR(w453, "Stop", w449) -> (w466:bool)
  }
  n234 = stacked-sequence {
    tunnel: [w485] -> w38
    tunnel: w39 -> [w485]
    frame #0 {
      n235 = local write "Stopped"(TRUE ("Stop")) -> ()
    }
  }
  n236 = Merge Errors(w38, w2, w8, w37, w13, w12, w11) -> (w45:errorcluster)
  n237 = call <vilib>:"IMAQdx Stop Acquisition.vi"("error in"=w45, "Session In"=w42) -> ("error out"=w51:errorcluster, "Session Out"=w52:T6)  [unwired: 8 out]
  n238 = call <vilib>:"IMAQdx Unconfigure Acquisition.vi"("error in"=w51, "Session In"=w52) -> ("error out"=w54:errorcluster, "Session Out"=w53:T6)  [unwired: 8 out]
  n239 = call <vilib>:"IMAQdx Close Camera.vi"("error in"=w54, "Session In"=w53) -> ("error out"=w41:errorcluster)  [unwired: 9 out]
  n240 = Release Queue(queue=w44, error in (no error)=w41) -> (error out=w40:errorcluster)  [unwired: 1 in, 2 out]
  n241 = for {
    shift-right: [w487] -> w32
    shift-left: w40 -> [w488]
    tunnel: w43 -> [w486] mode=indexing
    n242 = call "Imaq Dispose"("Image"=w486, "error in (no error)"=w488) -> ("error out"=w487:errorcluster)  [unwired: 4 in]
  }
  n243 = call <vilib>:"Simple Error Handler.vi"("error in (no error)"=w32) -> ()  [unwired: 4 in, 5 out]
